vi "Unflatten From String.vi"(7 "Type and Defaults":variant, 8 "error in (no error)":errorcluster, 10 "String":string, 11 "Deserializer in":refnum<class "JSON Deserializer.lvclass">) -> (0 "error out":errorcluster, 2 "Variant":variant, 3 "Deserializer out":refnum<class "JSON Deserializer.lvclass">)   [LabVIEW 2013, in "JKI JSON Serialization.lvlib" / "JSON Deserializer.lvclass"]
doc: "Converts a JSON formatted <b>String</b> to <b>Variant</b>. If <b>Type and Defaults</b> is provided, converts JSON string to the specified type if the type is compatible with the value of the JSON string. For any cluster element in Type and Defaults, the value of the element in Type and Default is used if element with the same name is not present in the JSON string."
uses:
  JSON Deserializer.lvclass
  JSON Parser/JSON Parser.lvclass
  <vilib>/Utility/VariantDataType/VariantType.lvlib
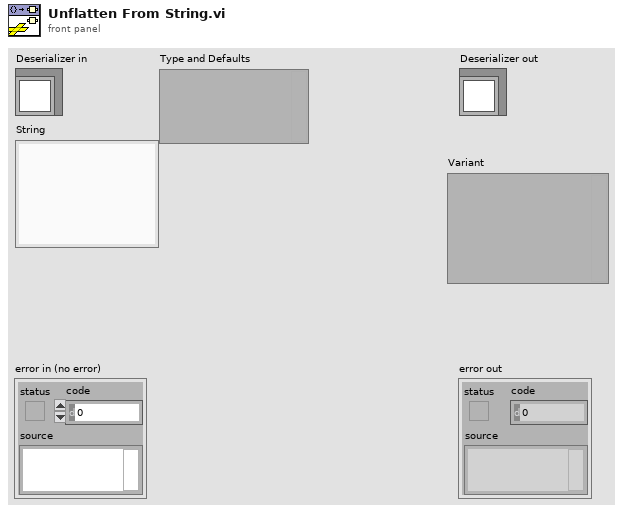
[diagram p1: front panel]
types:
  T1 = typedef "VariantType.lvlib/Type.ctl" = enum8{"Invalid Type", "Void", "I8", "I16", "I32", "I64", "U8", "U16", "U32", "U64", "Single Float", "Double Float", "Extended Float", "Single Complex", "Double Complex", "Extended Complex", "Enum U8", "Enum U16", "Enum U32", "Enum U64", "Single Float With Unit", "Double Float With Unit", "Extended Float With Unit", "Single Complex with Unit", "Double Complex with Unit", "Extended Complex with Unit", "Boolean", "String", "Path", "Picture", "Tag", "Array", "Cluster", "Variant", "LV Variant", "Waveform", "Timestamp", "Digital Waveform", "Digital Data", "ExpressData", "Refnum", "External Data", "VI", "Poly VI", "LabVIEW Class Instance", "Fixed Point"}
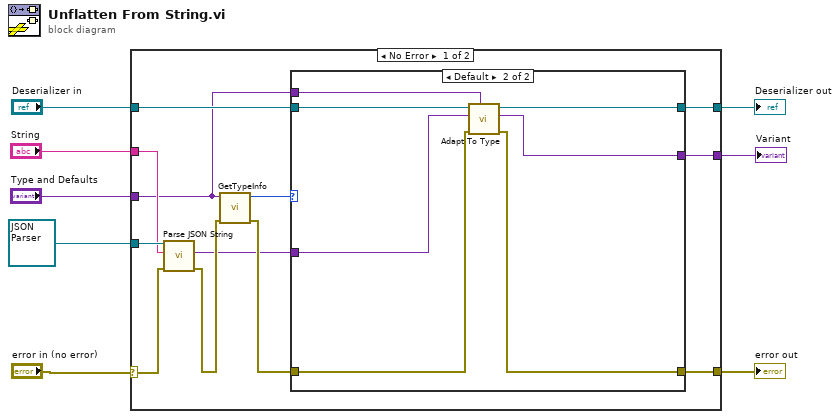
[diagram p0: block diagram]
diagram:
  n1 = case shown="No Error" "error in (no error)" {
    selector: "error in (no error)" -> [w19 w31]
    tunnel: "Deserializer in" -> [w13 w32]
    tunnel: refnum<class "JSON Parser.lvclass"> refnum ("Alpaca CLI Command Parser in") -> [w20 _]
    tunnel: "String" -> [w18 _]
    tunnel: [w15 w31] -> w4
    tunnel: "Type and Defaults" -> [w9 _]
    tunnel: [w12 w32] -> w2
    tunnel: [w11 _] -> w1
    frame No Error {
      n2 = call-dynamic "Parse JSON String.vi"("error in (no error)"=w19, "JSON String"=w18, "Alpaca CLI Command Parser in"=w20) -> ("error out"=w17:errorcluster, "Value"=w10:variant)  [unwired: 6 in, 1 out]
      n3 = call <vilib>:"GetTypeInfo.vi"("error in (no error)"=w17, "Variant"=w9) -> ("error out"=w14:errorcluster, "Type Enum"=w16:T1)  [unwired: 5 in, 3 out]
      n4 = case shown="Default" w16 {
        tunnel: [w22 w24] -> w15
        tunnel: w14 -> [w22 w25]
        tunnel: w13 -> [w23 w30]
        tunnel: [w23 w29] -> w12
        tunnel: [w21 w26] -> w11
        tunnel: w10 -> [w21 w27]
        tunnel: w9 -> [_ w28]
        frame "Void" {
        }
        frame Default {
          n5 = call "Adapt To Type.vi"("Type and Defaults"=w28, "error in (no error)"=w25, "Variant in"=w27, "Deserializer in"=w30) -> ("error out"=w24:errorcluster, "Variant out"=w26:variant, "Deserializer out"=w29:refnum<class "JSON Deserializer.lvclass">)  [unwired: 5 in]
        }
      }
    }
    frame Error {
    }
  }
  "error out" <- w4
  "Deserializer out" <- w2
  "Variant" <- w1
